vi "test classify error.vi"() -> (2 "errors unchanged":bool, 3 "classify as unknown":bool)   [LabVIEW 2013, in "TBM Tests.lvlib"]
uses:
  TBM Tests.lvlib
  runtime/TBM module execution interface.lvclass
  runtime/error classification.ctl
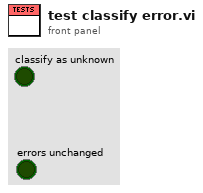
[diagram p1: front panel]
types:
  T1 = typedef "TBM module execution interface.lvclass/error classification.ctl" = enum16{"unknown", "none", "trivial", "recoverable", "critical"}
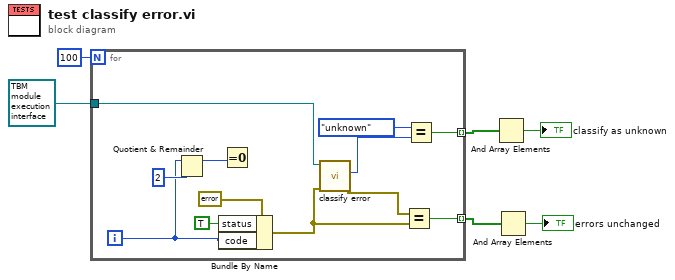
[diagram p0: block diagram]
diagram:
  n1 = for {
    N: 100 -> [_]
    tunnel: refnum<class "TBM module execution interface.lvclass"> refnum ("module") -> [w18]
    tunnel: [w15] -> w5 mode=indexing
    tunnel: [w7] -> w1 mode=indexing
    i -> [w10]
    n2 = Quotient & Remainder(x=w10, y=2) -> (x-y*floor(x/y)=w13:i32)  [unwired: 1 out]
    n3 = Bundle By Name(cluster=errorcluster {"status"=FALSE, "code"=0, "source"=""} ("error constant"), "status"=TRUE, "code"=w10) -> (w8:errorcluster)
    n4 = Equal To 0?(x=w13) -> ()  [unwired: 1 out]
    n5 = call-dynamic "classify error.vi"("error to classify"=w8, "module in"=w18) -> ("classified error"=w9:errorcluster, "error classification"=w17:T1)  [unwired: 7 in, 1 out]
    n6 = Equal?(x=w9, y=w8) -> (x = y?=w7:bool)
    n7 = Equal?(x=error_classification."unknown", y=w17) -> (x = y?=w15:bool)
  }
  n8 = And Array Elements(Boolean array=w5) -> (logical AND=→"classify as unknown":bool)
  n9 = And Array Elements(Boolean array=w1) -> (logical AND=→"errors unchanged":bool)
